vi "nirviSaturationMultiply.vi"(9 "x":i16, 13 "y":i16) -> (10 "x*y":i16, 18 "overflow":bool)   [LabVIEW 2017]
doc: "Computes the product of the inputs with configurable overflow handling and an optional overflow output."
panel:
  in  "operation":u16(ring)=2 items=["Add", "Sub", "Mult"]
  in  "Overflow terminal":bool
  in  "Lower Limit":i16=-128
  in  "Upper Limit":i16=127
  in  "Saturation":bool=TRUE
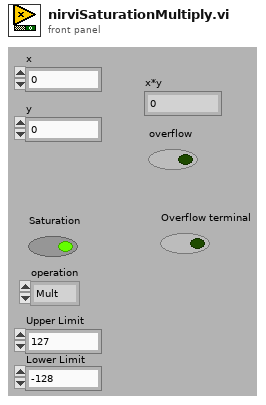
[diagram p1: front panel]
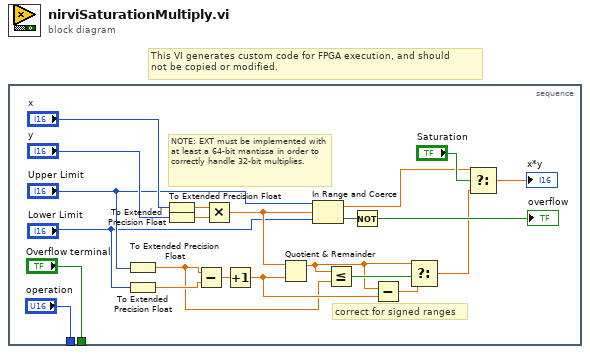
[diagram p0: block diagram]
diagram:
  # "This VI generates custom code for FPGA execution, and should\nnot be copied or modified."
  n1 = stacked-sequence {
    tunnel: ["Overflow terminal"] -> _
    tunnel: ["operation"] -> _
    frame #0 {
      # "NOTE: EXT must be implemented with at least a 64-bit mantissa in order to correctly handle 32-bit multiplies."
      # "correct for signed ranges"
      n2 = To Extended Precision Float(1:"Upper Limit") -> (0:w3:ext)
      n3 = To Extended Precision Float(1:"Lower Limit") -> (0:w10:ext)
      n4 = To Extended Precision Float(1:"x") -> (0:w18:ext)
      n5 = To Extended Precision Float(1:"y") -> (0:w19:ext)
      n6 = Subtract(x=w3, y=w10) -> (x-y=w9:ext)
      n7 = Multiply(x=w18, y=w19) -> (x*y=w13:ext)
      n8 = Increment(x=w9) -> (x+1=w4:ext)
      n9 = Quotient & Remainder(x=w13, y=w4) -> (x-y*floor(x/y)=w6:ext)  [unwired: 1 out]
      n10 = In Range and Coerce(upper limit="Upper Limit", x=w13, lower limit="Lower Limit") -> (coerced(x)=w16:ext, In Range?=w17:bool)
      n11 = Less Or Equal?(x=w6, y=w3) -> (x <= y?=w7:bool)
      n12 = Not(x=w17) -> (.not. x?=→"overflow":bool)
      n13 = Subtract(x=w6, y=w4) -> (x-y=w8:ext)
      n14 = Select(t=w6, s=w7, f=w8) -> (s? t:f=w5:ext)
      n15 = Select(t=w16, s="Saturation", f=w5) -> (s? t:f=→"x*y":ext)
    }
  }
